vi "DigitalWrite_MultiTask.vi"(2 "error in":errorcluster, 3 "input":bool[](array[boolean]), 4 "mutiTask":refnum<k21>) -> (0 "error out":errorcluster)   [LabVIEW 2015]
uses:
  <vilib>/DAQmx/write.llb/DAQmx Write (Digital 1D Bool NChan 1Samp 1Line).vi
  <vilib>/DAQmx/miscellaneous.llb/DAQmx Fill In Error Info.vi
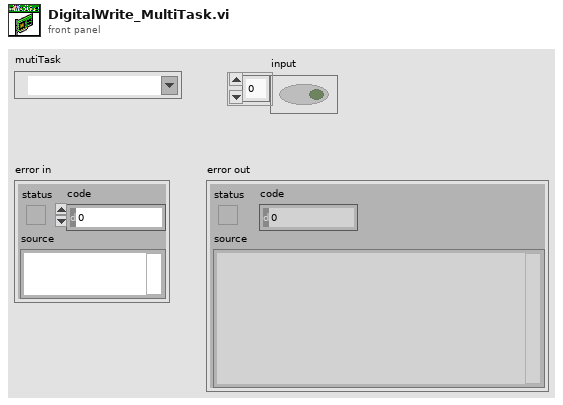
[diagram p1: front panel]
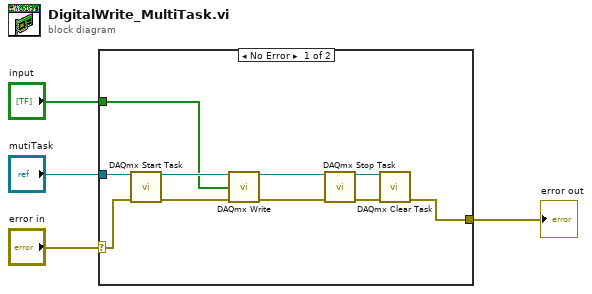
[diagram p0: block diagram]
diagram:
  n1 = case shown="No Error" "error in" {
    selector: "error in" -> [w5 w15]
    tunnel: "mutiTask" -> [w8 _]
    tunnel: "input" -> [w7 _]
    tunnel: [w6 w15] -> w1
    frame No Error {
      n2 = call <vilib>:"DAQmx Start Task.vi"("task/channels in"=w8, "error in"=w5) -> ("task out"=w14:refnum<k21>, "error out"=w13:errorcluster)  [unwired: 12 in]
      n3 = call-poly <vilib>:"DAQmx Write.vi"("task/channels in"=w14, "data"=w7, "error in"=w13) -> ("task out"=w12:refnum<k21>, "error out"=w11:errorcluster)  [unwired: 10 in, 1 out]
      n4 = call <vilib>:"DAQmx Stop Task.vi"("task/channels in"=w12, "error in"=w11) -> ("task out"=w9:refnum<k21>, "error out"=w10:errorcluster)  [unwired: 12 in]
      n5 = call <vilib>:"DAQmx Clear Task.vi"("task in"=w9, "error in"=w10) -> ("error out"=w6:errorcluster)  [unwired: 13 in]
    }
    frame Error {
    }
  }
  "error out" <- w1
